vi "WriteMessage.vi"(9 "HEX发送":bool, 10 "写入缓冲区":string, 11 "VISA资源名称":refnum<visa-resource-name>) -> (3 "VISA资源名称输出":refnum<visa-resource-name>)   [LabVIEW 2020]
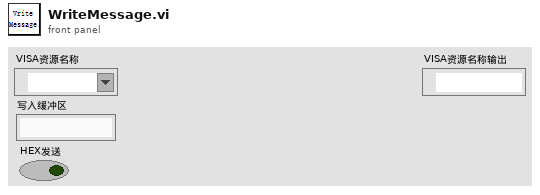
[diagram p1: front panel]
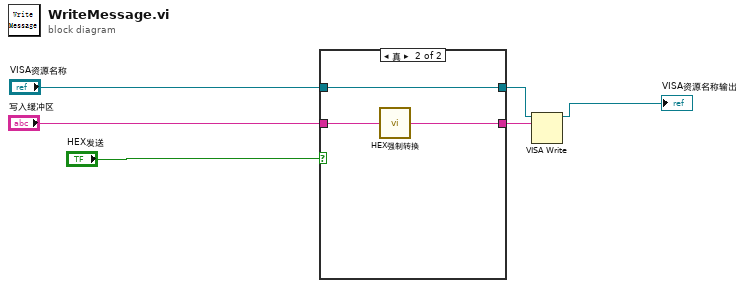
[diagram p0: block diagram]
diagram:
  n1 = case shown="真" "HEX发送" {
    tunnel: [w7 w11] -> w4
    tunnel: "VISA资源名称" -> [w7 w11]
    tunnel: "写入缓冲区" -> [w8 w10]
    tunnel: [w8 w9] -> w1
    frame False {
    }
    frame True {
      n2 = call "HEX强制转换.vi"("HexString"=w10) -> ("HEX"=w9:string)
    }
  }
  n3 = VISA Write(VISA resource name=w4, write buffer=w1) -> (VISA resource name out=→"VISA资源名称输出":refnum<visa-resource-name>)  [unwired: 1 in, 2 out]
